vi "Display_FGV.vi"(7 "Display_mods":T1, 8 "error in":errorcluster, 11 "variant":variant) -> (0 "error out":errorcluster, 3 "Base":picture)   [LabVIEW 2017]
uses:
  Display_mods.ctl
  Display_data.ctl
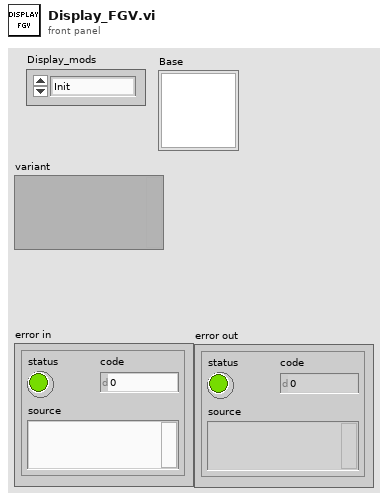
[diagram p1: front panel]
types:
  T1 = typedef "Display_mods.ctl" = enum16{"Init", "GetBase", "AddAster", "UpdateShip", "AddShoot", "DrawAll", "Clear", "Close"}
  T2 = typedef "Display_data.ctl" = cluster{"DisplayRef":refnum<vi>, "Shoots":cluster{"left":i16, "top":i16, "right":i16, "bottom":i16}[], "Asters":cluster{"rect":cluster{"left":i16, "top":i16, "right":i16, "bottom":i16}, "Fill":bool}[], "SpaceShip":cluster{"x":i16, "y":i16}[]}
  T3 = cluster{"rect":cluster{"left":i16, "top":i16, "right":i16, "bottom":i16}, "Fill":bool}
  T4 = cluster{"left":i16, "top":i16, "right":i16, "bottom":i16}
  T5 = cluster{"rect":cluster{"left":i16, "top":i16, "right":i16, "bottom":i16}, "Fill":bool}[]
  T6 = cluster{"left":i16, "top":i16, "right":i16, "bottom":i16}[]
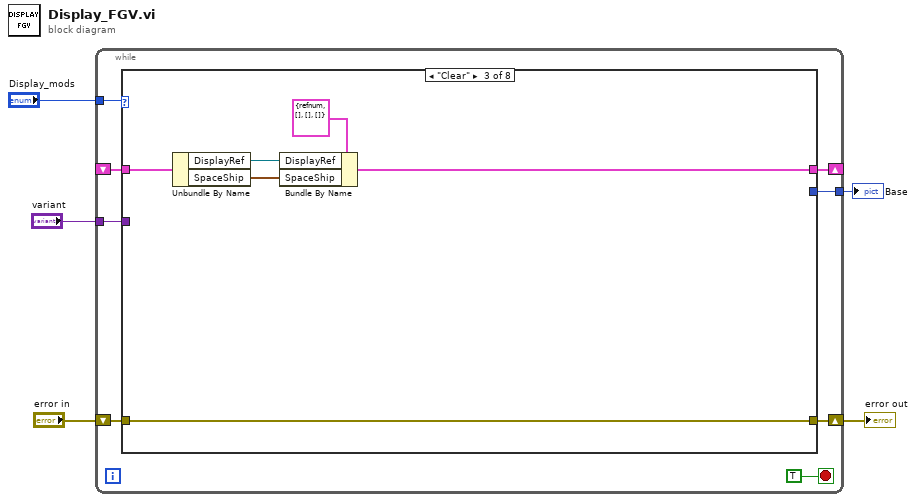
[diagram p0: block diagram]
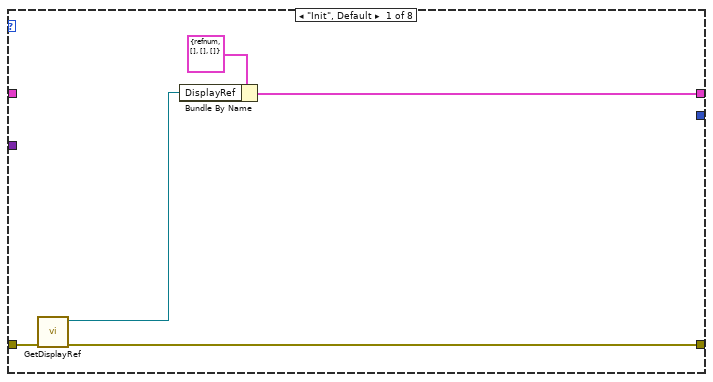
[diagram p2: hidden frame]
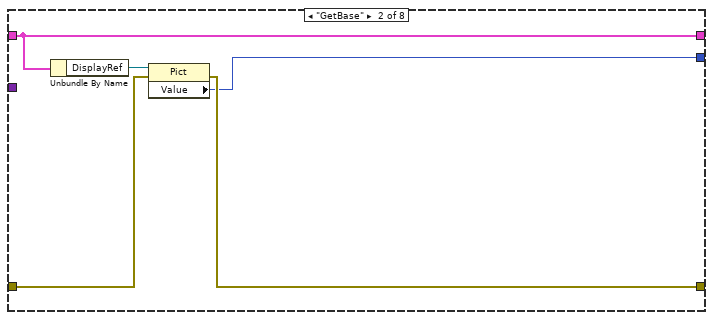
[diagram p3: hidden frame]
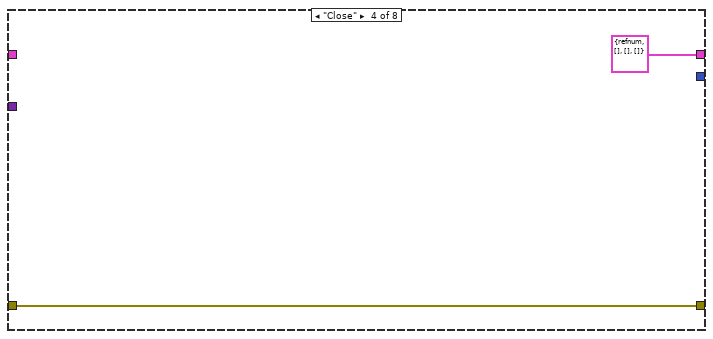
[diagram p4: hidden frame]
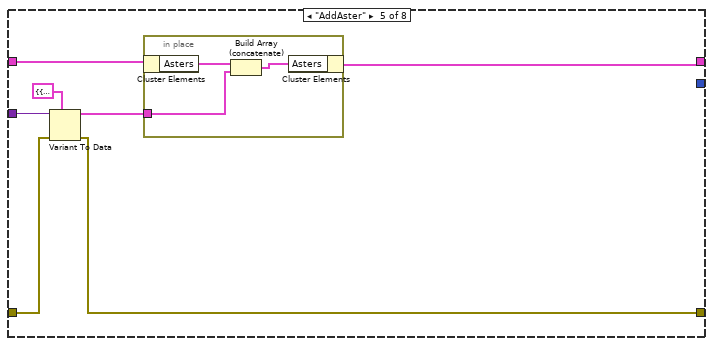
[diagram p5: hidden frame]
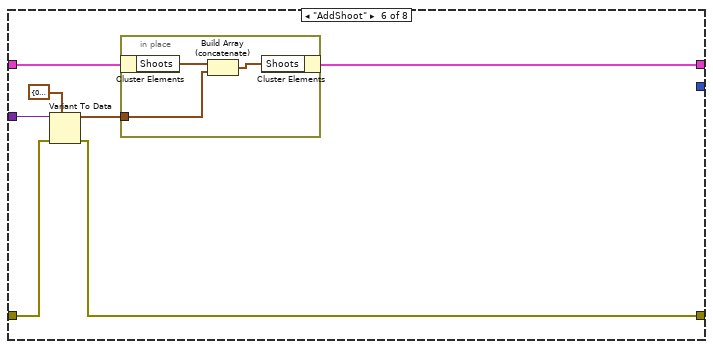
[diagram p6: hidden frame]
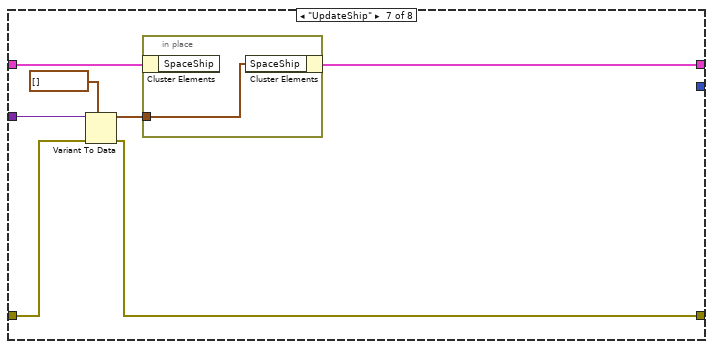
[diagram p7: hidden frame]
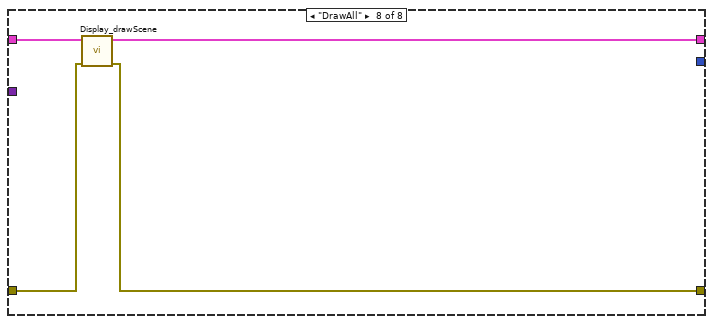
[diagram p8: hidden frame]
diagram:
  n1 = while {
    shift-right: [w10] -> w4
    shift-left: "error in" -> [w13]
    tunnel: "Display_mods" -> [w11]
    shift-right: [w8] -> _
    shift-left: _ -> [w9]
    tunnel: [w7] -> w2
    tunnel: "variant" -> [w6]
    stop <- TRUE stop-if-true
    n2 = case shown="\"Clear\"" w11 {
      tunnel: w13 -> [w18 w23 w25 w31 w37 w47 w57 w61]
      tunnel: [w17 w22 w25 w31 w32 w42 w52 w60] -> w10
      tunnel: w9 -> [_ w19 w29 _ w35 w45 w54 w63]
      tunnel: [w14 w19 w26 T2 {"DisplayRef"=refnum, "Shoots"=[], "Asters"=[], "SpaceShip"=[]} ("DisplayData") w33 w44 w53 w62] -> w8
      tunnel: [_ w21 _ _ _ _ _ _] -> w7
      tunnel: w6 -> [_ _ _ _ w38 w48 w58 _]
      frame "Init", Default {
        n3 = call "GetDisplayRef.vi"("error in"=w18) -> ("error out"=w17:errorcluster, "Picture out"=w15:refnum<vi>)  [unwired: 9 in]
        n4 = Bundle By Name(cluster=T2 {"DisplayRef"=refnum, "Shoots"=[], "Asters"=[], "SpaceShip"=[]} ("DisplayData"), "DisplayRef"=w15) -> (w14:T2)
      }
      frame "GetBase" {
        n5 = Unbundle By Name(w19) -> ("DisplayRef"=w20:refnum<vi>)
        n6 = property class="Pict"(reference=w20, error in=w23) -> (error out=w22:errorcluster, "Value"=w21:picture)  [unwired: 1 out]
      }
      frame "Clear" {
        n7 = Unbundle By Name(w29) -> ("DisplayRef"=w27:refnum<vi>, "SpaceShip"=w24:cluster{"x":i16, "y":i16}[])
        n8 = Bundle By Name(cluster=T2 {"DisplayRef"=refnum, "Shoots"=[], "Asters"=[], "SpaceShip"=[]} ("DisplayData"), "DisplayRef"=w27, "SpaceShip"=w24) -> (w26:T2)
      }
      frame "Close" {
      }
      frame "AddAster" {
        n9 = Variant To Data(error in=w37, type=T3 {"rect"={"left"=0, "top"=0, "right"=0, "bottom"=0}, "Fill"=FALSE} ("output cluster"), Variant=w38) -> (data=w34:T3, error out=w32:errorcluster)
        n10 = in-place {
          in-place-border: w34 -> [w40]
          n11 = in-place-cluster #1(w35) -> ("Asters"=w41:T5)
          n12 = Build Array (concatenate)(w41, w40) -> (w39:T5)
          n13 = in-place-cluster #1("Asters"=w39) -> (w33:T2)
        }
      }
      frame "AddShoot" {
        n14 = Variant To Data(error in=w47, type=T4 {"left"=0, "top"=0, "right"=0, "bottom"=0} ("rect"), Variant=w48) -> (data=w43:T4, error out=w42:errorcluster)
        n15 = in-place {
          in-place-border: w43 -> [w50]
          n16 = in-place-cluster #2(w45) -> ("Shoots"=w51:T6)
          n17 = Build Array (concatenate)(w51, w50) -> (w49:T6)
          n18 = in-place-cluster #2("Shoots"=w49) -> (w44:T2)
        }
      }
      frame "UpdateShip" {
        n19 = Variant To Data(error in=w57, type=cluster{"x":i16, "y":i16}[] [] ("SpaceshipLines"), Variant=w58) -> (data=w55:cluster{"x":i16, "y":i16}[], error out=w52:errorcluster)
        n20 = in-place {
          in-place-border: w55 -> [w59]
          n21 = in-place-cluster #3(w54) -> ()  [unwired: 1 out]
          n22 = in-place-cluster #3("SpaceShip"=w59) -> (w53:T2)
        }
      }
      frame "DrawAll" {
        n23 = call "Display_drawScene.vi"("error in"=w61, "DisplayData"=w63) -> ("error out"=w60:errorcluster, "DisplayData 2"=w62:T2)  [unwired: 8 in]
      }
    }
  }
  "error out" <- w4
  "Base" <- w2
